vi "uTTA_UploadFile.vi"(4 "error in":errorcluster, 5 "File Path":path, 6 "File Name":string, 7 "VISA Refnum in":refnum<visa-resource-name>) -> (0 "error out":errorcluster, 3 "VISA Refnum out":refnum<visa-resource-name>)   [LabVIEW 2021]
panel:
  out "Array":string[](array[string])
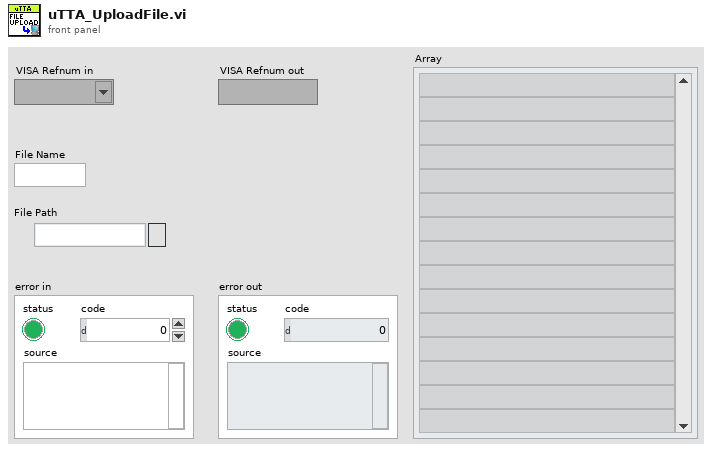
[diagram p1: front panel]
types:
  T1 = enum16{"open", "replace", "create", "open or create", "replace or create", "replace or create with confirmation"}
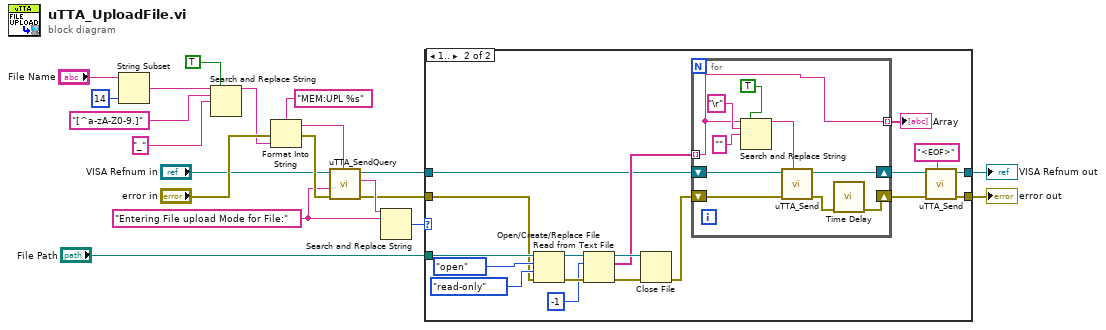
[diagram p0: block diagram]
diagram:
  w1 = "Entering File upload Mode for File:" ("search string")
  n1 = String Subset(string="File Name", length (rest)=14 ("length (rest)")) -> (substring=w10:string)  [unwired: 1 in]
  n2 = Search and Replace String(replace all?=TRUE ("replace all? (F)"), input string=w10, search string="[^a-zA-Z0-9.]", replace string="_" ("replace string (\"\")")) -> (result string=w9:string)  [unwired: 4 in, 3 out]
  n3 = Format Into String(format string="MEM:UPL %s", error in="error in", w9) -> (resulting string=w18:string, error out=w20:errorcluster)  [unwired: 1 in]
  n4 = call "uTTA_SendQuery.vi"("Send String"=w18, "error in (no error)"=w20, "Response Qualifier(\"\")"=w1, "VISA Refnum in"="VISA Refnum in") -> ("error out"=w5:errorcluster, "Received"=w8:string, "VISA Refnum out"=w6:refnum<visa-resource-name>)  [unwired: 5 in]
  n5 = Search and Replace String(input string=w8, search string=w1) -> (number of replacements=w7:i32)  [unwired: 6 in, 3 out]
  n6 = case shown="1.." w7 {
    tunnel: w6 -> [w22 w29]
    tunnel: w5 -> [w21 w37]
    tunnel: [w22 w25] -> w4
    tunnel: [w21 w24] -> w3
    tunnel: "File Path" -> [_ w40]
    frame 0, Default {
    }
    frame 1.. {
      n7 = Open/Create/Replace File(file path (use dialog)=w40, error in=w37, operation (0:open)=T1."open", access (0:read/write)=enum16{"read/write", "read-only", "write-only"}."read-only") -> (refnum out=w36:refnum<file>, error out=w35:errorcluster)  [unwired: 2 in, 1 out]
      n8 = Read from Text File(file (use dialog)=w36, count=-1, error in=w35) -> (refnum out=w32:refnum<file>, text=w30:string[], error out=w33:errorcluster)  [unwired: 1 in, 1 out]
      n9 = Close File(refnum=w32, error in=w33) -> (error out=w31:errorcluster)  [unwired: 1 out]
      n10 = for {
        tunnel: w30 -> [w41] mode=indexing
        shift-right: [w46] -> w27
        shift-left: w31 -> [w50]
        shift-right: [w47] -> w28
        shift-left: w29 -> [w48]
        tunnel: [w41] -> w23 mode=indexing
        n11 = Search and Replace String(replace all?=TRUE ("replace all? (F)"), input string=w41, search string="\r", replace string="" ("replace string (\"\")")) -> (result string=w42:string)  [unwired: 4 in, 3 out]
        n12 = call "uTTA_Send.vi"("Send String"=w42, "error in (no error)"=w50, "VISA Refnum in"=w48) -> ("error out"=w49:errorcluster, "VISA Refnum out"=w47:refnum<visa-resource-name>)  [unwired: 7 in]
        n13 = call "Time Delay"("error in (no error)"=w49) -> ("error out"=w46:errorcluster)  [unwired: 10 in]
      }
      "Array" <- w23
      n14 = call "uTTA_Send.vi"("Send String"="<EOF>", "error in (no error)"=w27, "VISA Refnum in"=w28) -> ("error out"=w24:errorcluster, "VISA Refnum out"=w25:refnum<visa-resource-name>)  [unwired: 7 in]
    }
  }
  "error out" <- w3
  "VISA Refnum out" <- w4
